vi "Test - Viterbi Algorithm.vi"() -> ()   [LabVIEW 2014, in "HMM.lvlib"]
uses:
  HMM.lvlib
panel:
  out "Hidden State Sequence":i32[](array[numeric])
  out "Partial Probalility":dbl[][](array[numeric])
  in  "Observed Sequence":i32[](array[numeric])
  in  "HMM Cluster":T1={"State transition matrix"=[[0.333, 0.333, 0.333], [0.333, 0.333, 0.333], [0.333, 0.333, 0.333]], "confusion matrix"=[[0.5, 0.5], [0.75, 0.25], [0.25, 0.75]], "Pi initial vector"=[0.333, 0.333, 0.333]}
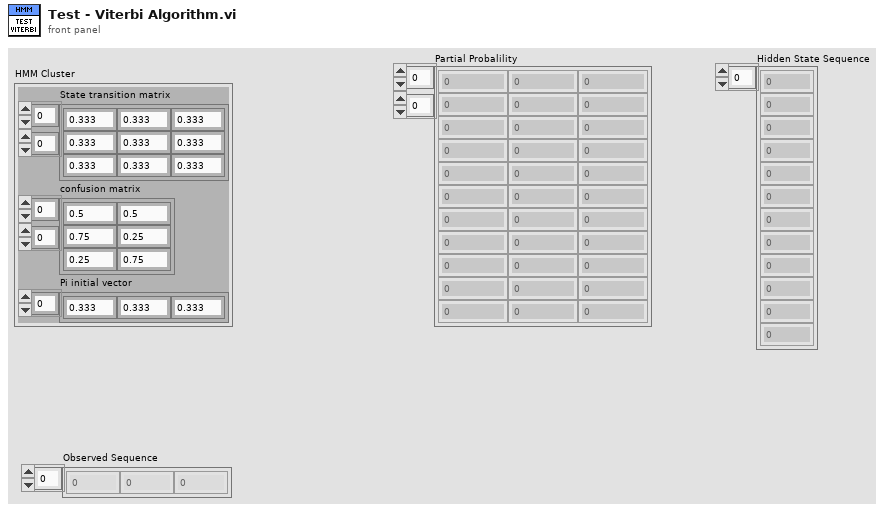
[diagram p1: front panel]
types:
  T1 = cluster{"State transition matrix":dbl[][], "confusion matrix":dbl[][], "Pi initial vector":dbl[]}
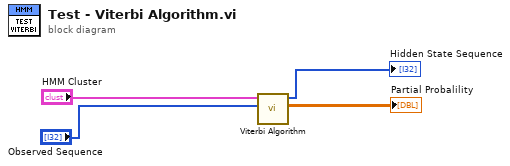
[diagram p0: block diagram]
diagram:
  n1 = call "Viterbi Algorithm.vi"("Observed Sequence"="Observed Sequence", "HMM Cluster"="HMM Cluster") -> ("Partial Probalility"=→"Partial Probalility":dbl[][], "Hidden State Sequence"=→"Hidden State Sequence":i32[])  [unwired: 8 in]
